vi "5492_RPMToTalonVelocity.vi"(11 "RPM":dbl) -> (3 "Talon Velocity":dbl)   [LabVIEW 2016]
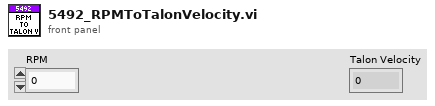
[diagram p1: front panel]
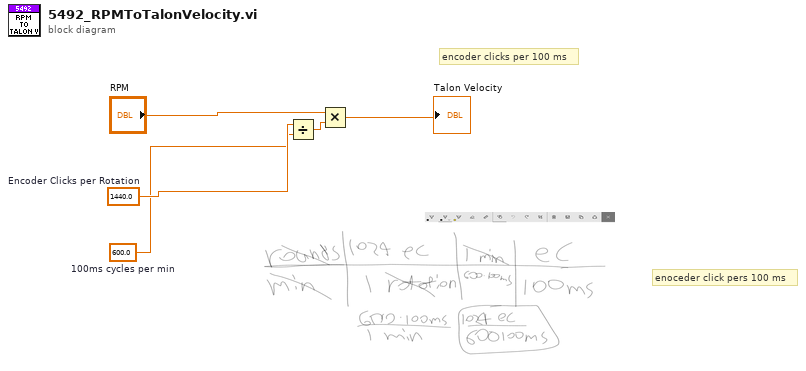
[diagram p0: block diagram]
diagram:
  w2 = 600.0  # 100ms cycles per min
  w3 = 1440.0  # Encoder Clicks per Rotation
  # "encoder clicks per 100 ms"
  # "enoceder click pers 100 ms"
  n1 = Divide(x=w3, y=w2) -> (x/y=w4:dbl)
  n2 = Multiply(x="RPM", y=w4) -> (x*y=→"Talon Velocity":dbl)
